vi "LIA_FPGA3a-PD Test-4vi.vi"() -> (1 "K Constant":fxp<+/-,32,16>, 2 "Nominal Freq":fxp<+/-,64,32>)   [LabVIEW 2012]
uses:
  <vilib>/rvi/DataTransferAndStorage/Container/Common/niFpgaContainerMetaDataKey.ctl
  <vilib>/rvi/DataTransferAndStorage/Container/Common/niFpgaContainerState.ctl
  <vilib>/rvi/DataTransferAndStorage/Container/Common/niFpgaDataTypeControl.ctl
  <vilib>/rvi/DataTransferAndStorage/Container/Common/niFpgaContainerImplementationControl.ctl
  <vilib>/rvi/DataTransferAndStorage/Container/Common/niFpgaContainerArbitrationOptionsControl.ctl
  <vilib>/rvi/DataTransferAndStorage/Container/Common/niFpgaTransferTypeControl.ctl
  <vilib>/rvi/DataTransferAndStorage/Container/Common/niFpgaContainerInitializationParameters.ctl
  <vilib>/rvi/Memory/Memory_Types/niFpgaMemoryInterfaceConfiguration.ctl
  <vilib>/rvi/FIFO/Fifo_Types/niFpgaFifoControlLogicControl.ctl
  <vilib>/Platform/TimedLoop/XDataNode/timing_clust.ctl
  <vilib>/Platform/TimedLoop/XDataNode/nitl_modes.ctl
  <vilib>/Platform/TimedLoop/XDataNode/wakeup.ctl
  <vilib>/rvi/FXPMathLib/basic elements/FxpIntAccumulator/subVIs/nifxpmath_IntAccumulator_SimConfig.ctl
  <vilib>/rvi/FXPMathLib/FxpSinAndCos/subVIs/nifxpmath_SinAndCos_SimConfig.ctl
  <vilib>/rvi/DataTransferAndStorage/Container/Common/niFpgaContainerGetUniqueNameForEmu.vi
  <vilib>/rvi/DataTransferAndStorage/Container/Common/niFpgaContainerSetEmuInfo.vi
  <vilib>/rvi/eio/common/nirviEmuReportErrorAndStop.vi
  <vilib>/rvi/FXPMathLib/basic elements/FxpIntAccumulator/simVIs/DllFxpIntAccumulator_sub.vi
  <vilib>/rvi/FXPMathLib/FxpSinAndCos/simVIs/DllFxpSinAndCosTemp_sub.vi
  <vilib>/rvi/eio/common/nirviEmuTemplateMethod_errors.vi
  <vilib>/rvi/Emulation/niFpgaSctlEmulationGetInTimedLoop.vi
  <vilib>/rvi/FIFO/Fifo_Resource/nirvififoEmulationSetSize.vi
  <vilib>/rvi/errors/niFpgaSetErrorForExecOnDevCompSimple.vi
  <vilib>/rvi/Emulation/niFpgaSctlEmulationFifoFullMgr.vi
  <vilib>/rvi/Emulation/niFpgaSctlEmulationResourceMgr.vi
  <vilib>/rvi/Emulation/niFpgaSctlEmulationRegisterWithScheduler.vi
  <vilib>/rvi/Emulation/niFpgaSctlEmulationScheduler.vi
  <vilib>/rvi/LocalResourceManager/LocalResourceManager.xnode
  <vilib>/Platform/TimedLoop/XDataNode/XDataNode.xnode
  <vilib>/rvi/FXPMathLib/basic elements/FxpIntAccumulator/XNode/nifxpmath_IntAccumulator.xnode
  <vilib>/rvi/FXPMathLib/FxpSinAndCos/XNode/nifxpmath_SinAndCos.xnode
  <vilib>/rvi/FXPMathLib/FxpMul/XNode/nifxpmath_Multiplier.xnode
  <vilib>/eio/EIONode/EIONode.xnode
  <vilib>/rvi/FXPMathLib/FxpInterpret/XNode/nifxpmath_Interpret.xnode
  <vilib>/rvi/DataTransferAndStorage/Container/XNode/niFpgaContainer.xnode
  <vilib>/rvi/FIFO/Fifo_Resource/nirvififoEmulationWrite.vi
  <vilib>/rvi/FIFO/Fifo_Resource/nirvififoEmulationRead.vi
  <vilib>/Platform/TimedLoop/XDataNode/XDNodeRunTimeDep.lvlib
  <vilib>/rvi/FXPMathLib/sim/FxpSim.dll
panel:
  in  "Z":fxp<+/-,64,32>
  in  "Voltage (V)":fxp<+/-,32,16>
  out "Numeric 2":fxp<+/-,64,32>
  out "Radians":fxp<+/-,14,5>
  out "Cos":fxp<+/-,14,2>
  out "Sin":fxp<+/-,14,2>
  in  "Period":u16=1000
  out "ticks":u16
  out "ref":i16 format="%.0x"
  out "sig":i16 format="%.0x"
  out "channelQ":i64
  out "channelI":i64
  out "f":fxp<+/-,32,0> format="%.32g"
  in  "start":bool
  in  "dec2":i16=1
  in  "K":fxp<+,16,0>=0.001007080078125
  in  "nominal freq":fxp<+,16,0>=0.010009765625
  in  "dec1":i16=1
  in  "stages":i8=1
  in  "stop":bool
  in  "decimation":i16=1024
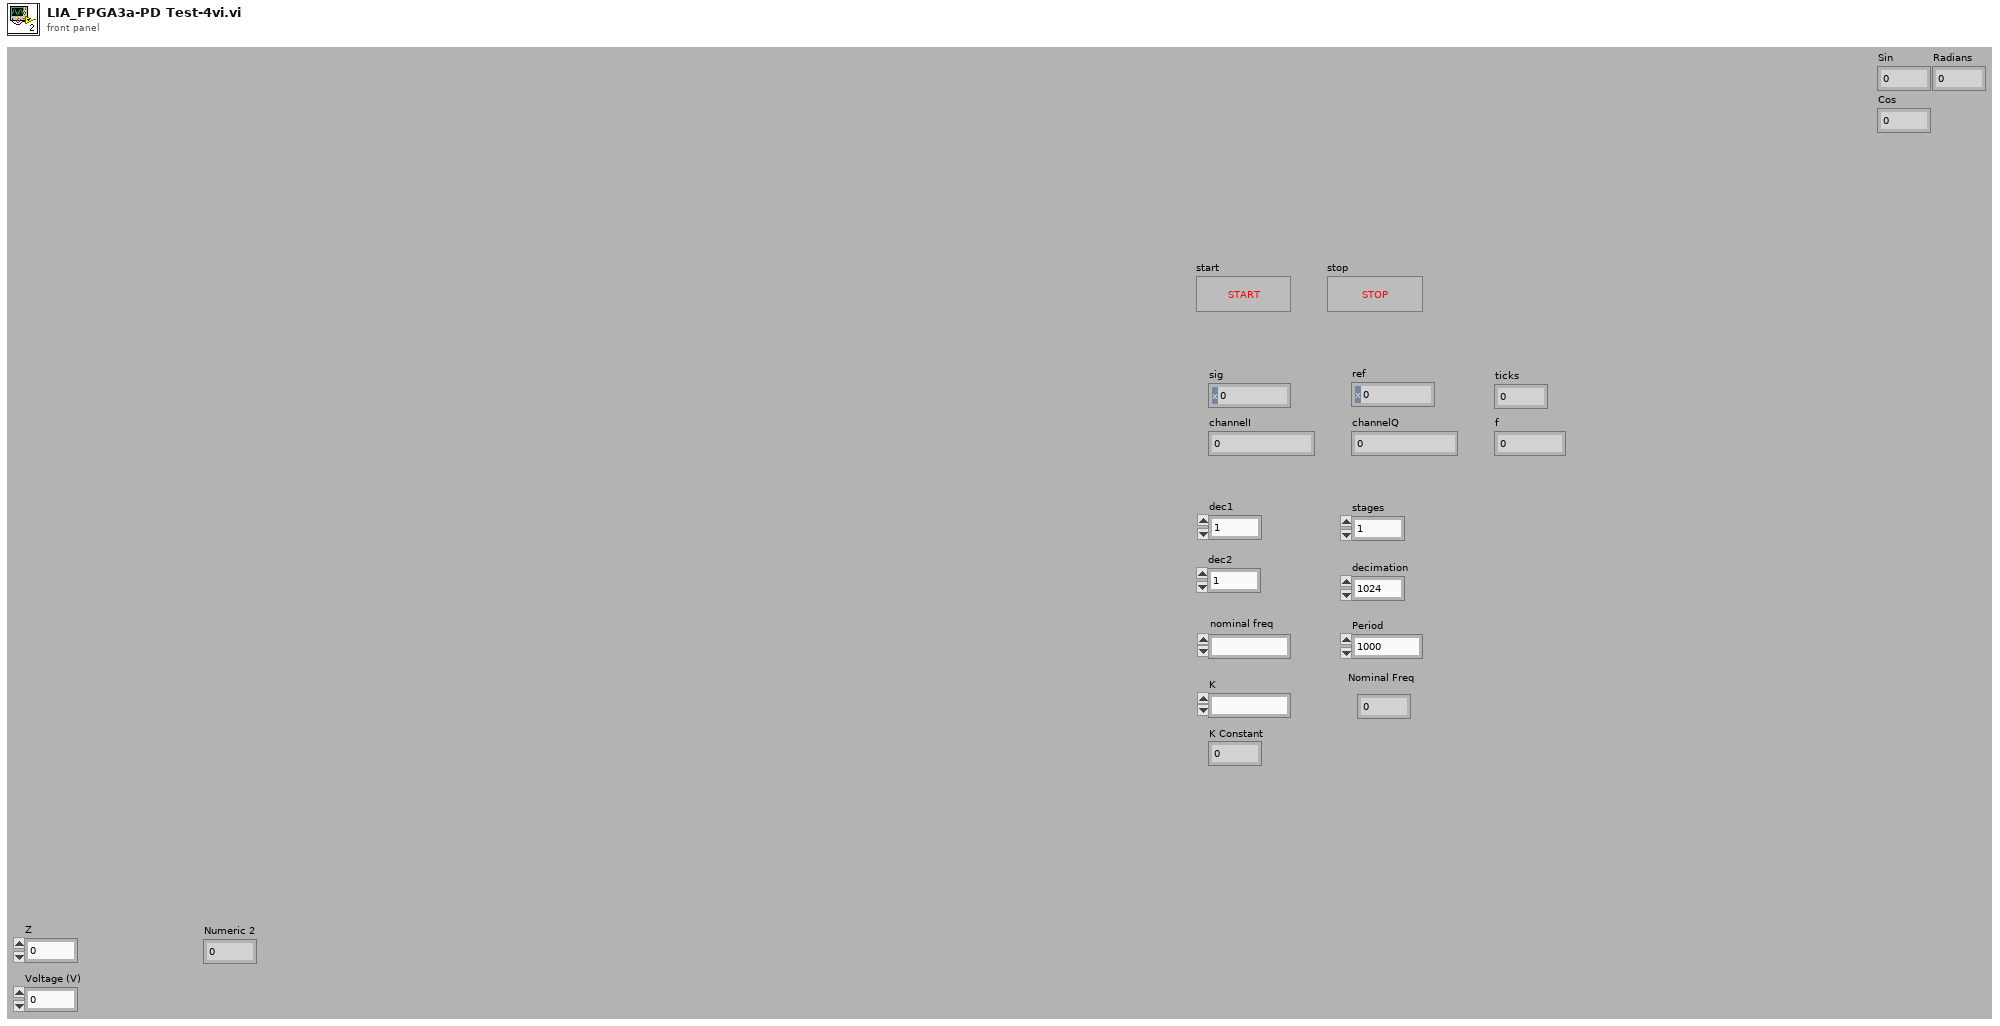
[diagram p1: front panel]
types:
  T1 = typedef "XDNodeRunTimeDep.lvlib/timing_clust.ctl" = cluster{"Expected End [f-1]":u64, "Actual End [f-1]":u64, "Finished Late? [f-1]":bool, "Expected End [i-1]":u64, "Actual End [i-1]":u64, "Finished Late? [i-1]":bool, "Expected Start [i]":u64, "Actual Start [i]":u64, "Expected Start [f]":u64, "Actual Start [f]":u64, "Source Name":string, "Structure Name":string, "Period":i64, "Deadline":i64, "Offset":i64, "Start":i64, "Priority":i32, "Timeout":i32, "Mode":T2, "Wakeup Reason":T3, "Error":errorcluster, "Source Type":string, "Secondary Source Type":string, "Global End Time":u64, "Global Start Time":u64, "Frame Duration":u64, "Iteration Duration":u64, "Assigned CPU":i32, "I/O Scan Engine Mode":u32}
  T2 = typedef "XDNodeRunTimeDep.lvlib/nitl_modes.ctl" = enum32{"No Change", "Process missed periods, maintain original phase", "Discard missed periods, maintain original phase", "Process missed periods, ignore original phase", "Discard missed periods, ignore original phase"}
  T3 = typedef "XDNodeRunTimeDep.lvlib/wakeup.ctl" = enum32{"Normal", "Aborted", "Asynchronous wakeup", "Timing source error", "Timed loop error", "Timeout"}
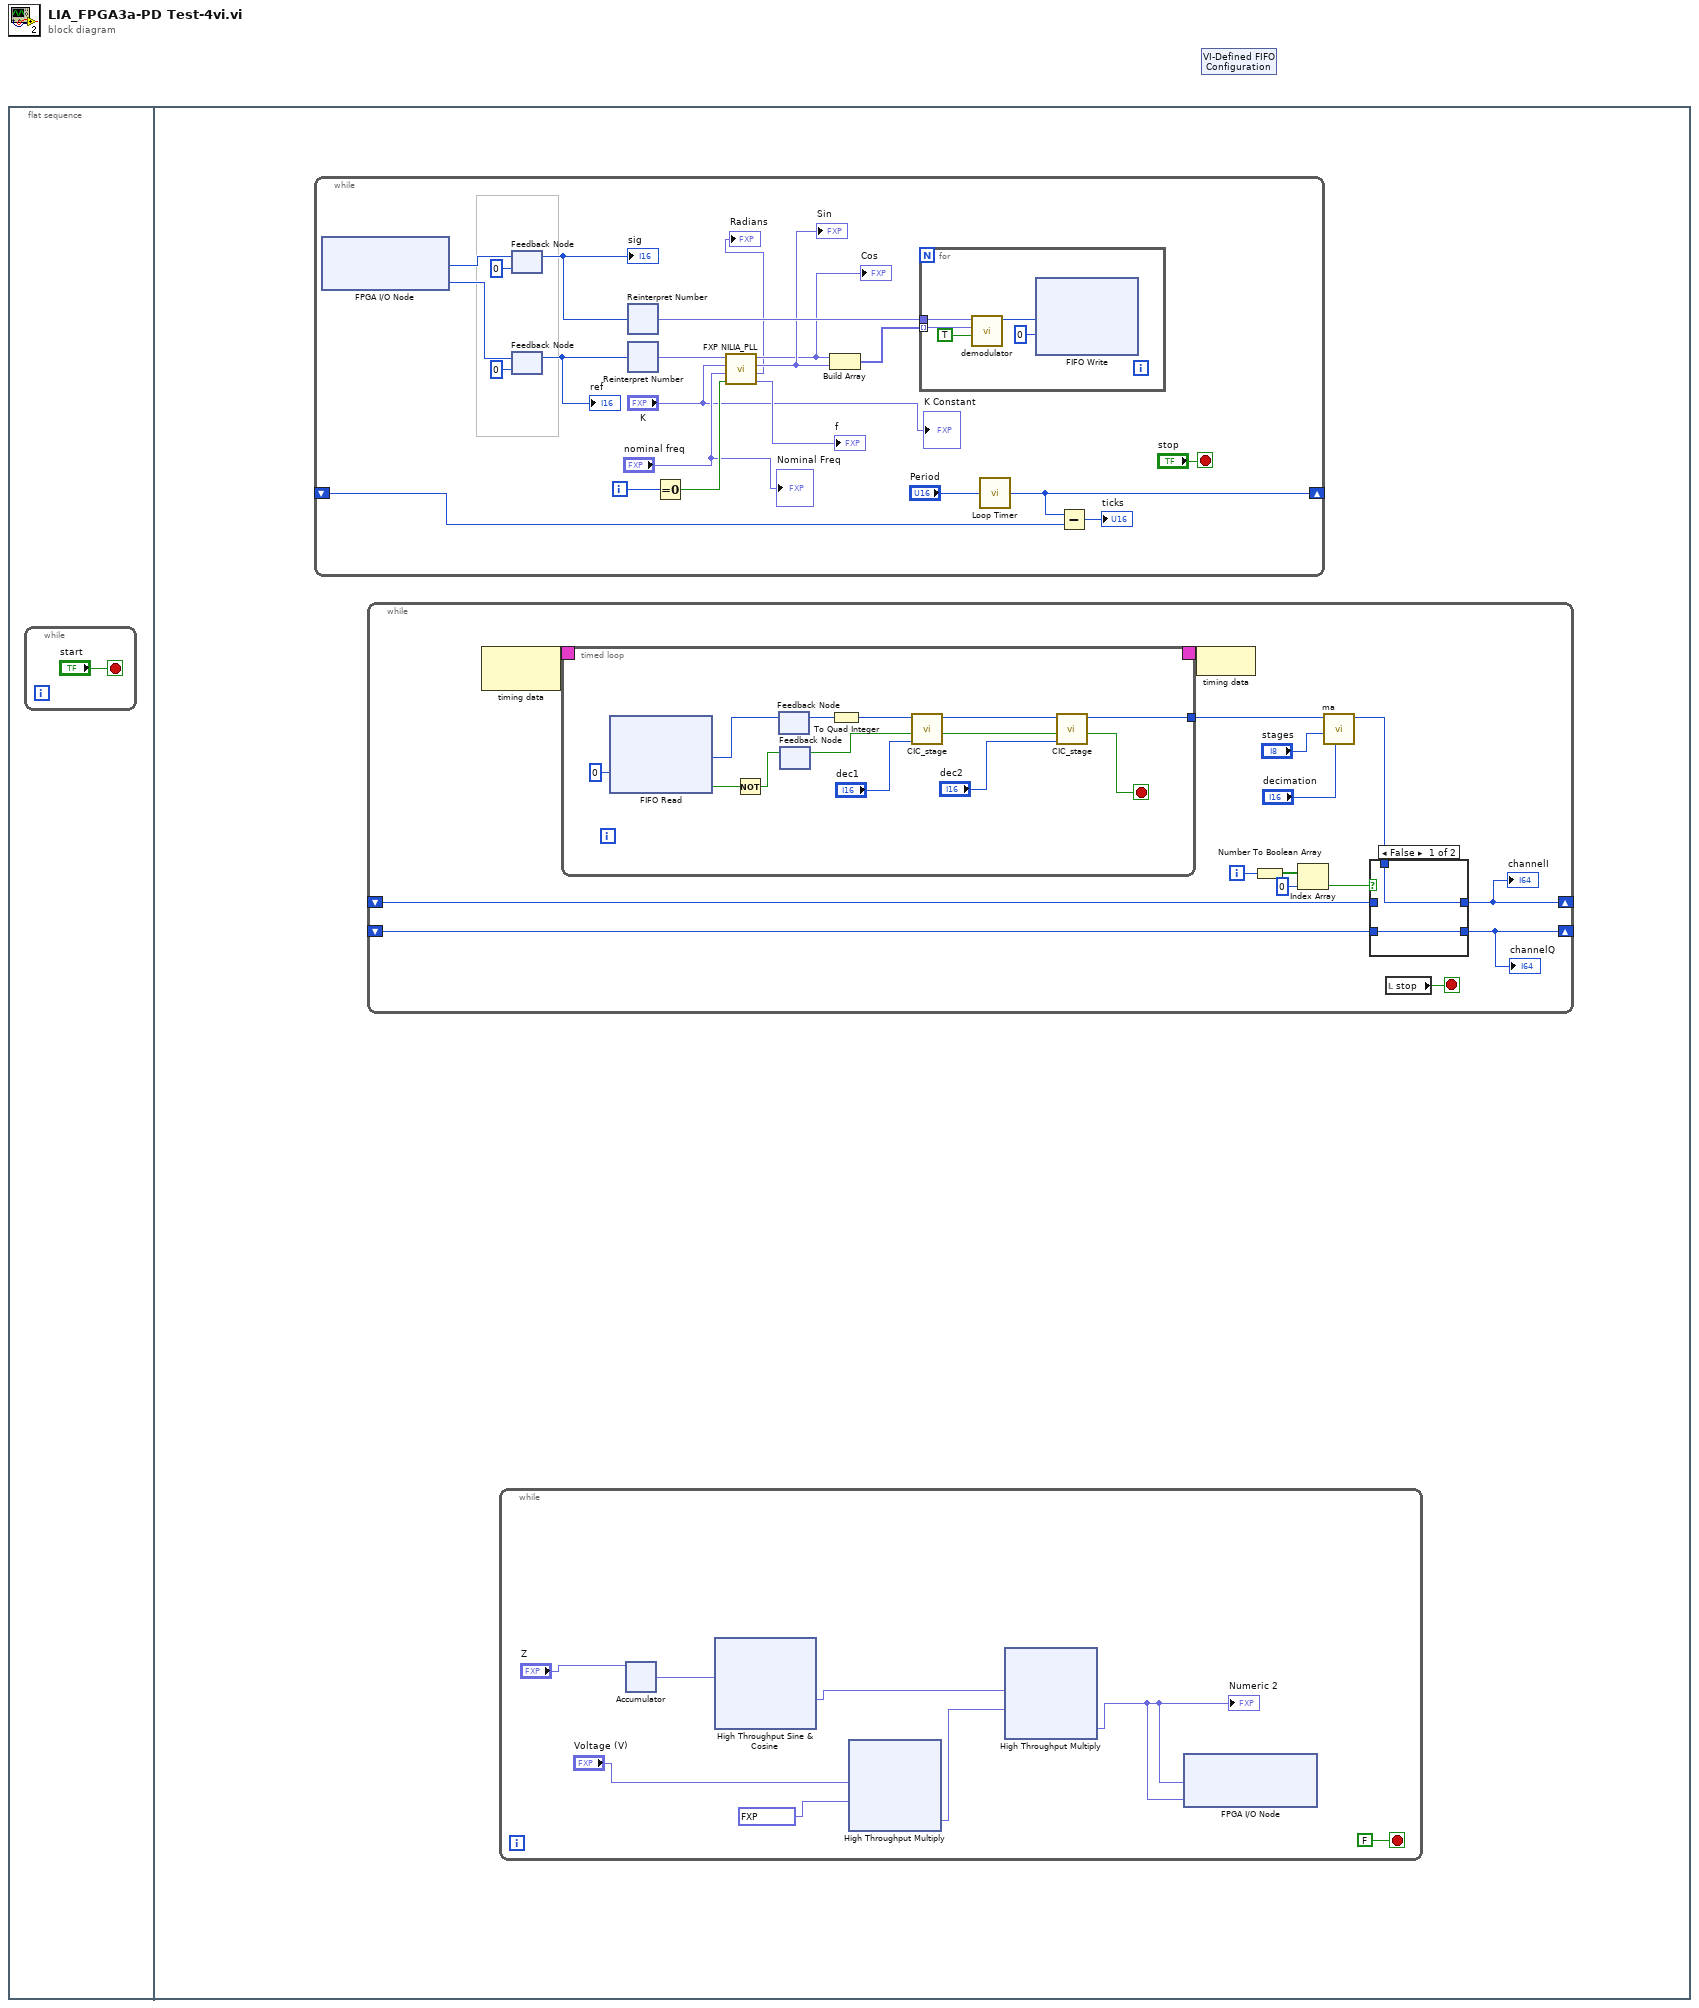
[diagram p0: block diagram]
diagram:
  n1 = flat-sequence {
    frame #0 {
      n2 = while {
        stop <- "start" stop-if-true
      }
    }
    frame #1 {
      n3 = while {
        shift-right: [w85] -> _
        shift-left: _ -> [w84]
        i -> [w88]
        stop <- "stop" stop-if-true
        n4 = xnode "FPGA I/O Node"() -> ("Connector0/AI6"=w78:i16, "Connector0/AI7"=w75:i16)  [unwired: 2 in, 2 out]
        n5 = feedback #1(i16 0 ("y")) -> (w77:i16)
        "sig" <- w77
        n6 = feedback-in #1(w78) -> ()
        n7 = feedback #2(i16 0 ("z [I32.1]")) -> (w76:i16)
        "ref" <- w76
        n8 = feedback-in #2(w75) -> ()
        n9 = xnode "Reinterpret Number"("x"=w77) -> ("y"=w81:fxp<+/-,16,1>)
        n10 = xnode "Reinterpret Number"("x"=w76) -> ("y"=w74:fxp<+/-,16,1>)
        n11 = Equal To 0?(x=w88) -> (x = 0?=w72:bool)
        n12 = call "FXP NILIA_PLL.vi"("reset?"=w72, "norminal freq [U16.0]"="nominal freq", "alpha [U16.0]"="K", "x[I16.1]"=w74) -> ("f"=→"f":fxp<+/-,32,0>, "z [I32.1]"=→"Radians":fxp<+/-,32,1>, "sin(z)"=w69:fxp<+/-,16,2>, "cos(z)"=w68:fxp<+/-,16,2>)  [unwired: 4 in]
        "Sin" <- w69
        "Cos" <- w68
        n13 = Build Array(w68, w69) -> (w82:fxp<+/-,16,2>[])
        n14 = for {
          tunnel: w81 -> [w91]
          tunnel: w82 -> [w89] mode=indexing
          n15 = call "demodulator.vi"("New Data"=TRUE, "ref"=w89, "signal"=w91) -> ("x*y"=w92:i32)  [unwired: 8 out]
          n16 = xnode ("FIFO Write")("Element"=w92, "Timeout"=0) -> ()  [unwired: 1 in, 2 out]
        }
        n17 = call "Loop Timer"("Count(Ticks)"="Period") -> ("Tick Count(Ticks)"=w85:u16)
        n18 = Subtract(x=w85, y=w84) -> (x-y=→"ticks":u16)
        "Nominal Freq" <- "nominal freq"
        "K Constant" <- "K"
      }
      n19 = while {
        shift-right: [w95] -> _
        shift-left: _ -> [w97]
        shift-right: [w94] -> _
        shift-left: _ -> [w96]
        i -> [w102]
        stop <- w104 stop-if-true
        n20 = node-c288() -> (w108:T1)  [unwired: 1 out]
        n21 = timed-loop {
          timing: w108 -> [_]
          timing-out: [_] -> w107
          tunnel: [w116] -> w103
          stop <- w115 stop-if-true
          n22 = xnode ("FIFO Read")("Timeout"=0) -> ("Element"=w123:i32, "Timed Out?"=w122:bool)  [unwired: 1 in, 1 out]
          n23 = Not(x=w122) -> (.not. x?=w121:bool)
          n24 = feedback-in #3(w123) -> ()
          n25 = feedback #3() -> (w125:i32)  [unwired: 1 out]
          n26 = feedback-in #4(w121) -> ()
          n27 = feedback #4() -> (w119:bool)  [unwired: 1 out]
          n28 = To Quad Integer(1:w125) -> (0:w120:i64)
          n29 = call "CIC_stage.vi"("decimate factor"="dec1", "New Data"=w119, "input"=w120) -> ("Data Ready"=w117:bool, "output"=w118:i64)  [unwired: 7 out]
          n30 = call "CIC_stage.vi"("decimate factor"="dec2", "New Data"=w117, "input"=w118) -> ("Data Ready"=w115:bool, "output"=w116:i64)  [unwired: 7 out]
        }
        n31 = node-c288(w107) -> ()
        n32 = Number To Boolean Array(number=w102) -> (Boolean array=w101:bool[])
        n33 = Index Array "Index Array"(array=w101, index=0) -> (element=w99:bool)
        n34 = call "ma.vi"("decimate"="decimation", "stages"="stages", "input"=w103) -> ("output"=w98:i64)  [unwired: 8 out]
        n35 = case shown="False" w99 {
          tunnel: w98 -> [w110 w112]
          tunnel: [w110 w111] -> w95
          tunnel: [w109 w112] -> w94
          tunnel: w97 -> [_ w111]
          tunnel: w96 -> [w109 _]
          frame False {
          }
          frame True {
          }
        }
        "channelI" <- w95
        "channelQ" <- w94
        n36 = local read "stop"() -> (w104:bool)
      }
      n37 = while {
        stop <- FALSE stop-if-true
        n38 = xnode "Accumulator"("x"="Z") -> ("s"=w7:fxp<+/-,64,32>)  [unwired: 4 in, 1 out]
        n39 = xnode "High Throughput Sine & Cosine"("x (pi)"=w7) -> ("sin(x)"=w5:fxp<+/-,16,2>)  [unwired: 1 out]
        n40 = xnode ("High Throughput Multiply")("x"="Voltage (V)", "y"=fxp<+,16,12> 3276.8125) -> ("x*y"=w6:fxp<+/-,48,28>)
        n41 = xnode ("High Throughput Multiply")("x"=w5, "y"=w6) -> ("x*y"=w2:fxp<+/-,64,30>)
        "Numeric 2" <- w2
        n42 = xnode "FPGA I/O Node"("Connector0/AO2"=w2, "Connector0/AO1"=w2) -> ()  [unwired: 2 in, 2 out]
      }
    }
  }
  n43 = xnode "VI-Defined FIFO Configuration"() -> ()  [unwired: 1 out]
